vi "Teleop Operator Controls.vi"(7 "Call Context":T1=enum."Stop", 9 "Intaking":bool, 10 "Driver Agree To Shoot? (F)":bool, 11 "Match Info":T2={"Autonomous Elapsed Seconds"=0.0, "TeleOp Elapsed Seconds"=5.101, "Disabled Elapsed Seconds"=19.516, "Visited Autonomous"=FALSE, "Visited TeleOp"=TRUE, "Visited Disabled"=TRUE, "Autonomous Settings"={"Autonomous Style"=enum."Independent", "VI Refnum"=refnum}}) -> (3 "Operator Ready To Shoot?":bool)   [LabVIEW 2019]
uses:
  <vilib>/Rock Robotics/WPI/DriverStation/WPI_DriverStationMatch Info.ctl
  <vilib>/Rock Robotics/WPI/DriverStation/WPI_DriverStationDerivedRobotMode.ctl
  Typedef/XBox Axis.ctl
  Typedef/XBox Buttons.ctl
  Typedef/XBox POV.ctl
  <vilib>/Rock Robotics/WPI/Utilities/WPI_GetSetVariantRefNum.vi
panel:
  in  "LL Jog Amount":dbl
  in  "Hood Jog Amount Fast":dbl=0.5
  in  "Fast Jog Degress/frame":dbl=1.0
  in  "Jog Holdtime (ms)":u32=300
  in  "270 Hood Angle":dbl
  in  "180 Hood Angle":dbl
  in  "90 Hood Angle":dbl=10.0
  in  "0 Hood Angle":dbl=20.0
  in  "270 Angle":dbl
  in  "180 Angle":dbl
  in  "90 Angle":dbl=90.0
  in  "0 Angle":dbl
  in  "Hood Jog Amount":dbl=0.5
  in  "Jog Degrees":dbl=1.0
  in  "WoD Deadband":dbl=0.3
  in  "WoD Speed Factor":dbl=0.4
  in  "Uptake Speed":dbl=1.0 format="%#_13g"
  in  "Shooter Shoot RPM":dbl=7000.0
  in  "Shooter Idle RPM":dbl=2000.0
  in  "Turret Stick Deadband":dbl=0.9
  # "0"
  # "TURRET"
  # "HOOD"
  # "Joystick"
  # "90"
  # "270"
  # "180"
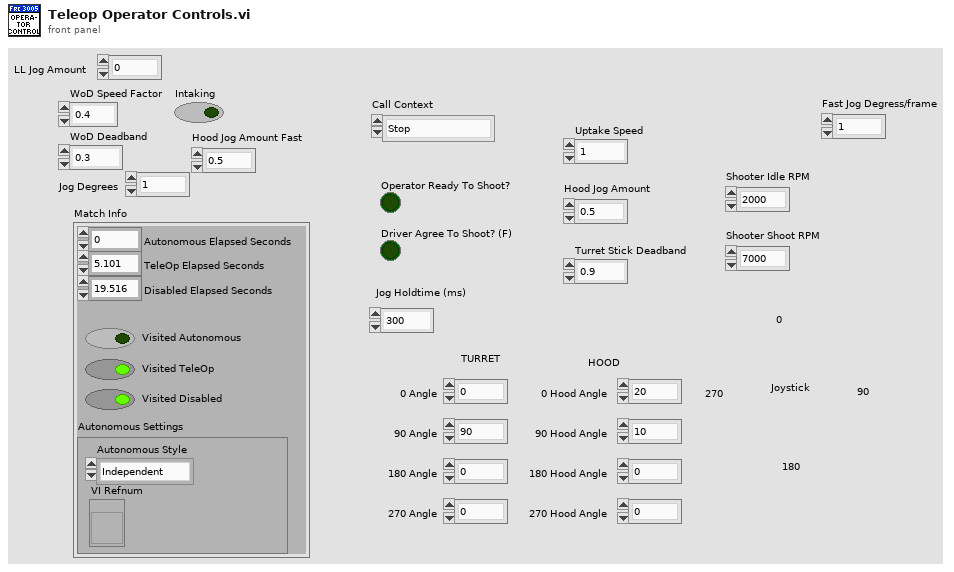
[diagram p1: front panel]
types:
  T1 = typedef "WPI_DriverStationDerivedRobotMode.ctl" = enum16{"Init", "Execute", "Stop"}
  T2 = typedef "WPI_DriverStationMatch Info.ctl" = cluster{"Autonomous Elapsed Seconds":dbl, "TeleOp Elapsed Seconds":dbl, "Disabled Elapsed Seconds":dbl, "Visited Autonomous":bool, "Visited TeleOp":bool, "Visited Disabled":bool, "Autonomous Settings":cluster{"Autonomous Style":enum16{"Iterative", "Independent"}, "VI Refnum":refnum<vi>}}
  T3 = typedef "XBox Axis.ctl" = enum16{"Left X", "Left Y", "Left Trigger", "Right Trigger", "Right X", "Right Y"}
  T4 = typedef "XBox Buttons.ctl" = enum16{"A", "B", "X", "Y", "Left Bumper", "Right Bumper", "Back", "Start", "Left Joystick", "Right Joystick"}
  T5 = typedef "XBox POV.ctl" = enum16{"Center", "Top", "Top Right", "Center Right", "Bottom Right", "Bottom", "Bottom Left", "Center Left", "Top Left"}
  T6 = typedef "WPI_JoystickDevRef.ctl" = cluster{"Device":T7}
  T7 = typedef "WPI_JoystickDeviceEnum.ctl" = enum16{"USB 0", "USB 1", "USB 2", "USB 3", "USB 4", "USB 5"}
  T8 = typedef "Command Status Info.ctl" = cluster{"Name":string, "Status":T9, "notifier out":T10}
  T9 = typedef "Completion Status.ctl" = enum16{"Successful", "Aborted", "Incomplete"}
  T10 = typedef "Completion Notifier.ctl" = refnum<notifier>
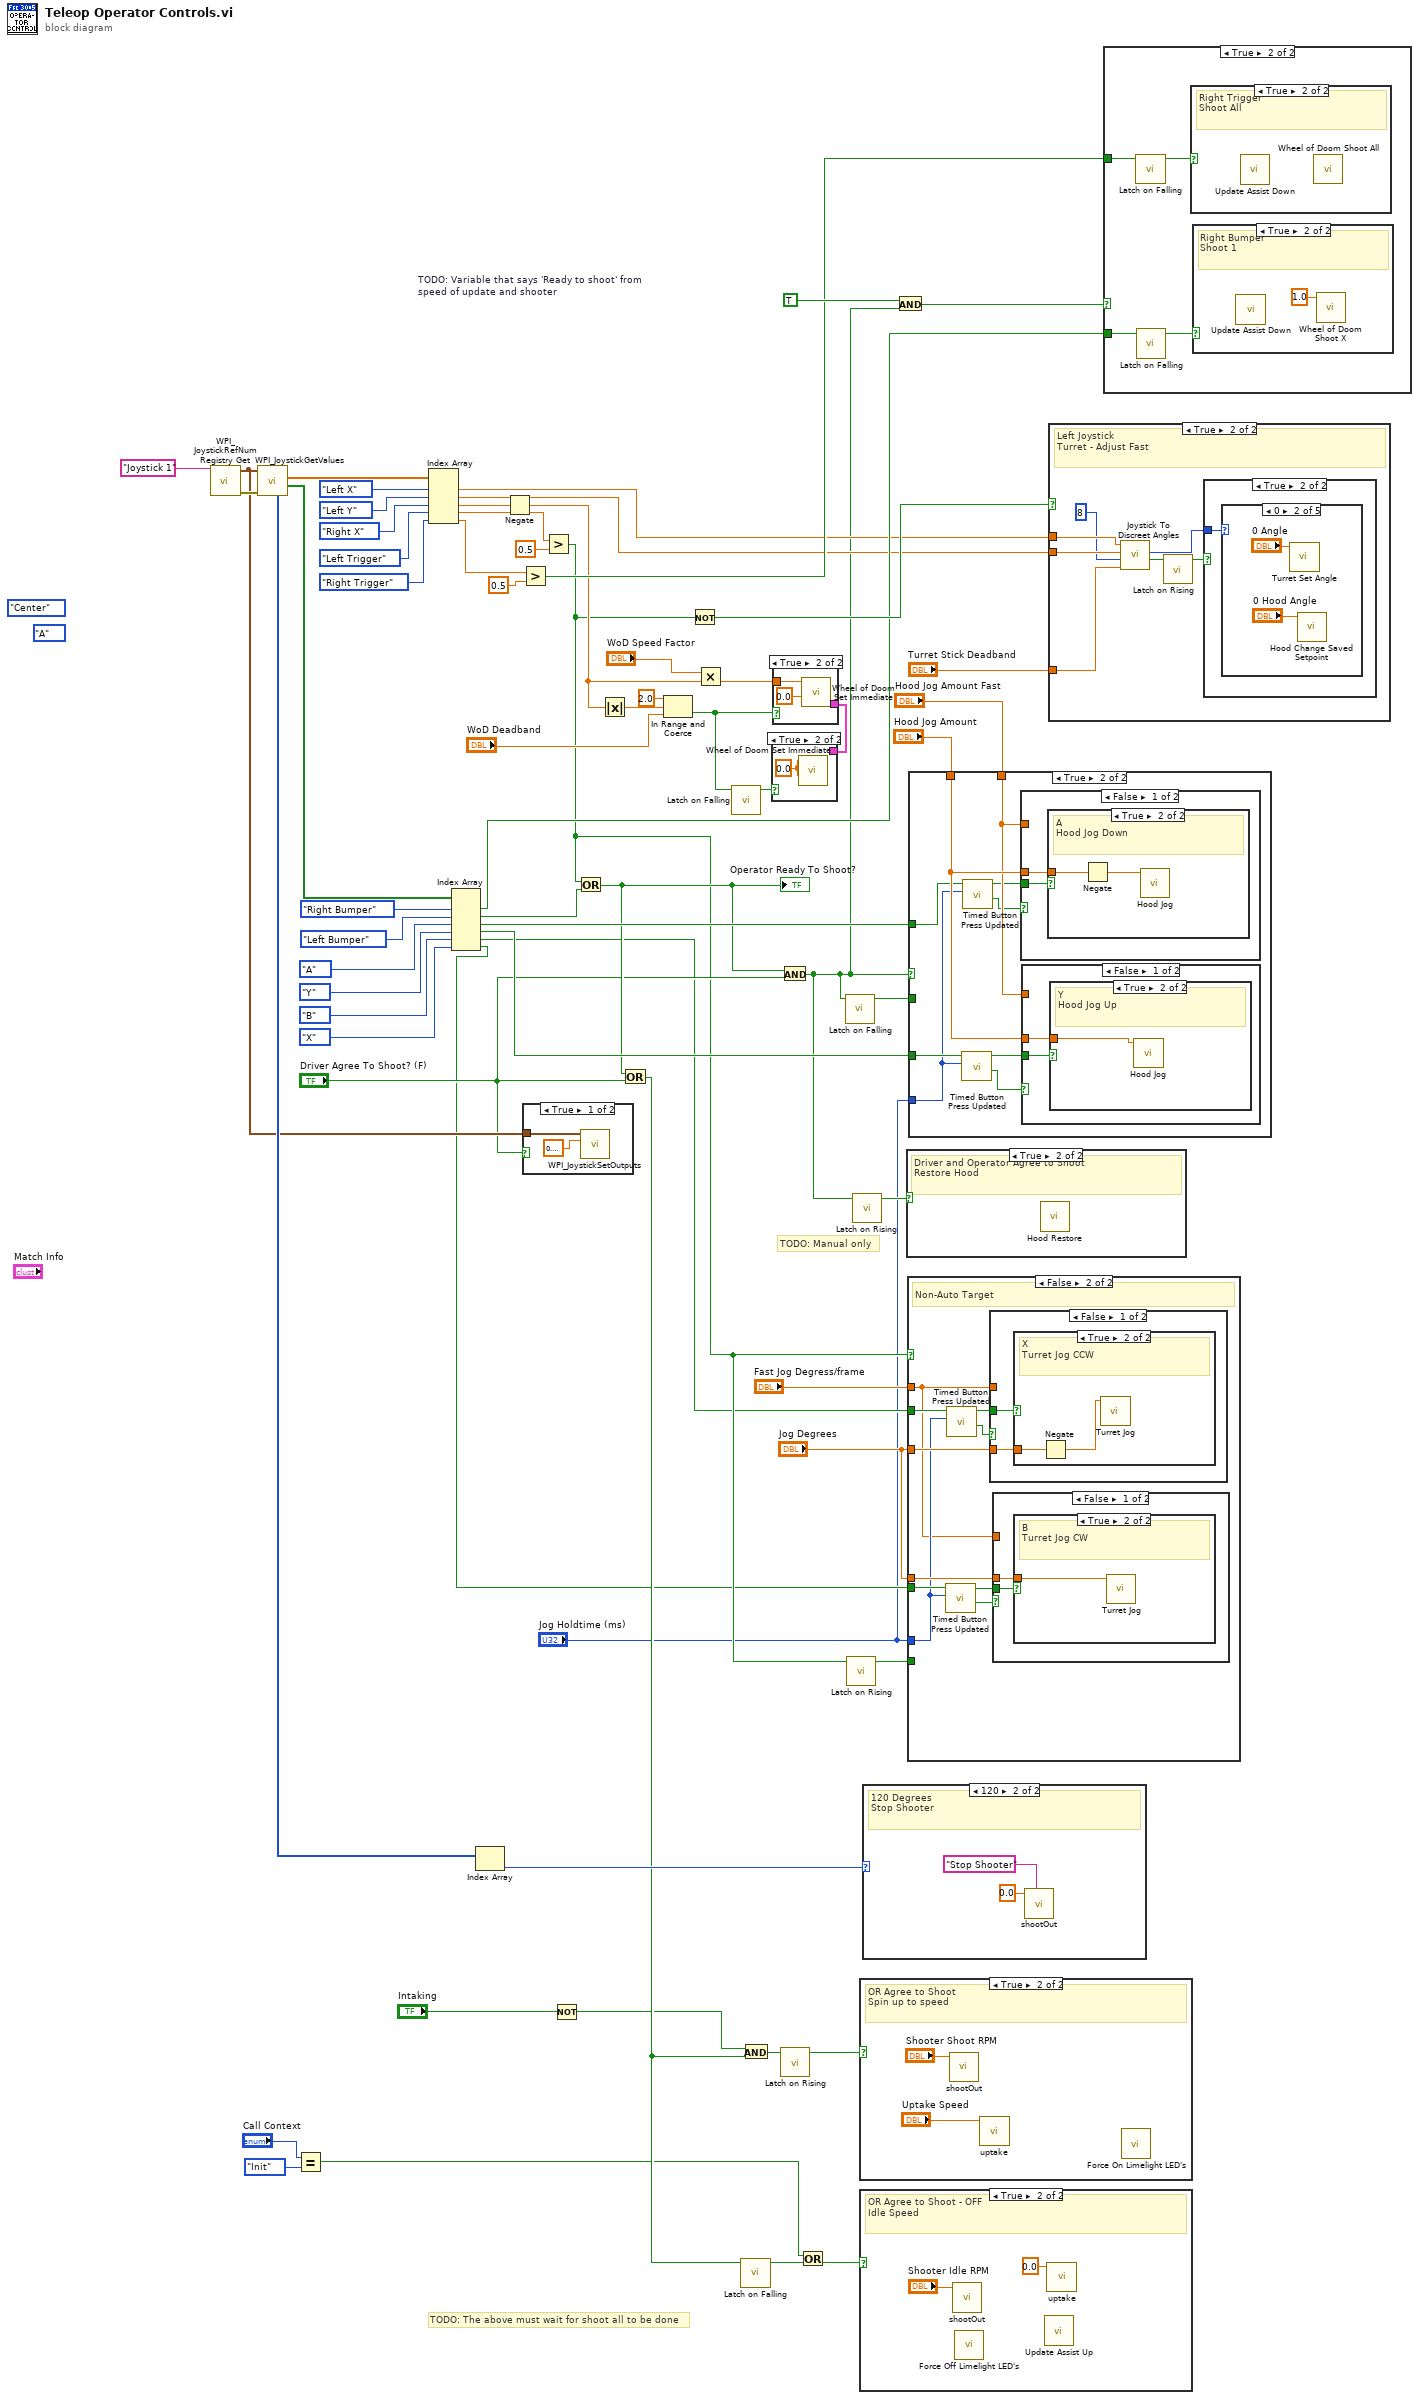
[diagram p0: block diagram]
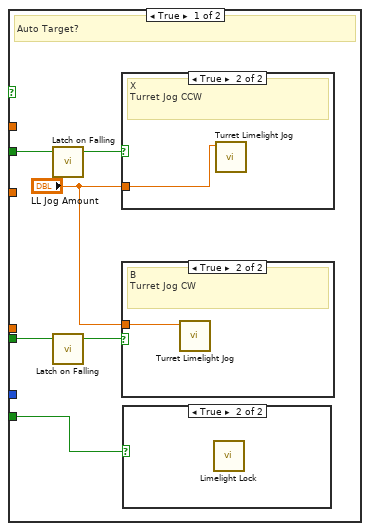
[diagram p3: hidden frame]
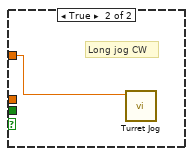
[diagram p8: hidden frame]
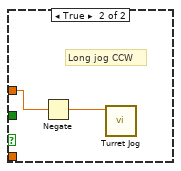
[diagram p10: hidden frame]
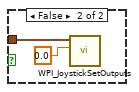
[diagram p11: hidden frame]
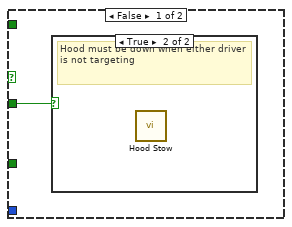
[diagram p19: hidden frame]
diagram:
  w44 = TRUE  # TODO: Variable that says 'Ready to shoot' from speed of update and shooter
  (unwired) XBox_Buttons."A" ("Enum 2")
  (unwired) XBox_POV."Center" ("Enum")
  # "TODO: Manual only"
  # "TODO: The above must wait for shoot all to be done"
  n1 = call <vilib>:"WPI_JoystickRefNum Registry Get.vi"("refnum name"="Joystick 1") -> ("error out"=w66:errorcluster, "JoystickDevRef"=w23:T6)  [unwired: 9 in]
  n2 = call <vilib>:"WPI_JoystickGetValues.vi"("error in (no error)"=w66, "JoystickDevRef"=w23) -> ("Buttons"=w64:bool[], "Axes"=w65:dbl[], "POVs"=w54:i16[])  [unwired: 5 in, 2 out]
  n3 = Equal?(x="Call Context", y=WPI_DriverStationDerivedRobotMode."Init") -> (x = y?=w8:bool)
  n4 = Index Array(array=w65, index #1=XBox_Axis."Left X" ("Enum 3"), index #2=XBox_Axis."Left Y" ("Enum 3"), index #3=XBox_Axis."Right X" ("Enum 3"), index #4=XBox_Axis."Left Trigger" ("Enum 3"), index #5=XBox_Axis."Right Trigger" ("Enum 3")) -> (element #1=w34:dbl, element #2=w33:dbl, element #3=w28:dbl, element #4=w50:dbl, element #5=w40:dbl)
  n5 = Index Array(array=w64, index #1=XBox_Buttons."Right Bumper" ("Enum 2"), index #2=XBox_Buttons."Left Bumper" ("Enum 2"), index #3=XBox_Buttons."A" ("Enum 2"), index #4=XBox_Buttons."Y" ("Enum 2"), index #5=XBox_Buttons."B" ("Enum 2"), index #6=XBox_Buttons."X" ("Enum 2")) -> (element #1=w42:bool, element #2=w48:bool, element #3=w61:bool, element #4=w56:bool, element #5=w7:bool, element #6=w6:bool)
  n6 = Index Array(array=w54) -> (element=w53:i16)  [unwired: 1 in]
  n7 = Negate(x=w28) -> (-x=w24:dbl)
  n8 = Greater?(x=w40, y=0.5) -> (0:w38:bool)
  n9 = case shown="True" "Driver Agree To Shoot? (F)" {
    tunnel: w23 -> [w69 w71]
    frame True {
      n10 = call <vilib>:"WPI_JoystickSetOutputs.vi"("Left Rumble"=sgl 0.3, "JoystickDevRef"=w69) -> ()  [unwired: 8 in, 2 out]
    }
    frame False {
      n11 = call <vilib>:"WPI_JoystickSetOutputs.vi"("Left Rumble"=sgl 0.0, "JoystickDevRef"=w71) -> ()  [unwired: 8 in, 2 out]
    }
  }
  n12 = Greater?(x=w50, y=0.5) -> (0:w19:bool)
  n13 = Not(x="Intaking") -> (.not. x?=w13:bool)
  n14 = Or(x=w19, y=w48) -> (x .or. y?=w37:bool)
  "Operator Ready To Shoot?" <- w37
  n15 = Absolute Value(x=w24) -> (abs(x)=w25:dbl)
  n16 = Or(x=w37, y="Driver Agree To Shoot? (F)") -> (x .or. y?=w15:bool)
  n17 = In Range and Coerce(upper limit=2.0, x=w25, lower limit="WoD Deadband") -> (In Range?=w27:bool)  [unwired: 1 out]
  n18 = Not(x=w19) -> (.not. x?=w46:bool)
  n19 = Multiply(x="WoD Speed Factor", y=w24) -> (x*y=w32:dbl)
  n20 = call <vilib>:"Latch on Falling.vi"("Boolean in"=w27) -> ("Boolean out"=w26:bool)  [unwired: 4 in]
  n21 = call <vilib>:"Latch on Falling.vi"("Boolean in"=w15) -> ("Boolean out"=w36:bool)  [unwired: 4 in]
  n22 = And(x=w13, y=w15) -> (x .and. y?=w16:bool)
  n23 = case shown="True" w27 {
    tunnel: w32 -> [_ w74]
    tunnel: [_ w72] -> w1
    frame False {
    }
    frame True {
      n24 = call "Wheel of Doom Set Immediate.vi"("Deadband Value"=0.0, "Setpoint"=w74) -> ("Command Info Out"=w72:T8)  [unwired: 9 in]
    }
  }
  n25 = case shown="True" w26 {
    tunnel: w1 -> [_ _]
    frame False {
    }
    frame True {
      w75 = 0.0 ("Deadband Value")
      n26 = call "Wheel of Doom Set Immediate.vi"("Deadband Value"=w75, "Setpoint"=w75) -> ()  [unwired: 9 in, 1 out]
    }
  }
  n27 = And(x=w37, y="Driver Agree To Shoot? (F)") -> (x .and. y?=w2:bool)
  n28 = call <vilib>:"Latch on Rising.vi"("Boolean in"=w16) -> ("Boolean out"=w35:bool)  [unwired: 4 in]
  n29 = Or(x=w8, y=w36) -> (x .or. y?=w11:bool)
  n30 = call <vilib>:"Latch on Falling.vi"("Boolean in"=w2) -> ("Boolean out"=w47:bool)  [unwired: 4 in]
  n31 = call <vilib>:"Latch on Rising.vi"("Boolean in"=w19) -> ("Boolean out"=w18:bool)  [unwired: 4 in]
  n32 = call <vilib>:"Latch on Rising.vi"("Boolean in"=w2) -> ("Boolean out"=w17:bool)  [unwired: 4 in]
  n33 = case shown="True" w35 {
    frame False {
    }
    frame True {
      # "OR Agree to Shoot\nSpin up to speed"
      n34 = call "shootOut.vi"("Setpoint"="Shooter Shoot RPM") -> ()  [unwired: 10 in, 1 out]
      n35 = call "uptake.vi"("Setpoint"="Uptake Speed") -> ()  [unwired: 10 in, 1 out]
      n36 = call "Force On Limelight LED's.vi"() -> ()  [unwired: 10 in, 1 out]
    }
  }
  n37 = case shown="True" w11 {
    frame False {
    }
    frame True {
      # "OR Agree to Shoot - OFF\nIdle Speed"
      n38 = call "shootOut.vi"("Setpoint"="Shooter Idle RPM") -> ()  [unwired: 10 in, 1 out]
      n39 = call "Force Off Limelight LED's.vi"() -> ()  [unwired: 10 in, 1 out]
      n40 = call "Update Assist Up.vi"() -> ()  [unwired: 11 in, 1 out]
      n41 = call "uptake.vi"("Setpoint"=0.0) -> ()  [unwired: 10 in, 1 out]
    }
  }
  n42 = case shown="120" w53 {
    frame 0, Default {
    }
    frame 120 {
      # "120 Degrees\nStop Shooter"
      n43 = call "shootOut.vi"("Description"="Stop Shooter", "Setpoint"=0.0) -> ()  [unwired: 9 in, 1 out]
    }
  }
  n44 = And(x=w44, y=w2) -> (x .and. y?=w45:bool)
  n45 = case shown="True" w17 {
    frame False {
    }
    frame True {
      # "Driver and Operator Agree to Shoot\nRestore Hood"
      n46 = call "Hood Restore.vi"() -> ()  [unwired: 11 in, 1 out]
    }
  }
  n47 = case shown="False" w19 {
    tunnel: w7 -> [w87 w95]
    tunnel: w6 -> [w86 w97]
    tunnel: "Jog Degrees" -> [_ w99]
    tunnel: "Jog Degrees" -> [_ w98]
    tunnel: w18 -> [w85 _]
    tunnel: "Jog Holdtime (ms)" -> [_ w93]
    tunnel: "Fast Jog Degress/frame" -> [_ w92]
    frame True {
      # "Auto Target?"
      n48 = call <vilib>:"Latch on Falling.vi"("Boolean in"=w87) -> ("Boolean out"=w82:bool)  [unwired: 4 in]
      n49 = call <vilib>:"Latch on Falling.vi"("Boolean in"=w86) -> ("Boolean out"=w83:bool)  [unwired: 4 in]
      n50 = case shown="True" w82 {
        tunnel: "LL Jog Amount" -> [_ w89]
        frame False {
        }
        frame True {
          # "X\nTurret Jog CCW"
          n51 = call "Turret Limelight Jog.vi"("Jog Amount"=w89) -> ()  [unwired: 11 in]
        }
      }
      n52 = case shown="True" w83 {
        tunnel: "LL Jog Amount" -> [_ w88]
        frame False {
        }
        frame True {
          # "B\nTurret Jog CW"
          n53 = call "Turret Limelight Jog.vi"("Jog Amount"=w88) -> ()  [unwired: 11 in]
        }
      }
      n54 = case shown="True" w85 {
        frame False {
        }
        frame True {
          n55 = call "Limelight Lock.vi"() -> ()  [unwired: 11 in, 1 out]
        }
      }
    }
    frame False {
      # "Non-Auto Target"
      n56 = call "Timed Button Press Updated.vi"("Holdtime (ms)"=w93, "Input"=w97) -> ("Long Press Held"=w91:bool, "Quick Press"=w96:bool)  [unwired: 6 in, 2 out]
      n57 = call "Timed Button Press Updated.vi"("Holdtime (ms)"=w93, "Input"=w95) -> ("Long Press Held"=w90:bool, "Quick Press"=w94:bool)  [unwired: 6 in, 2 out]
      n58 = case shown="False" w90 {
        tunnel: w99 -> [w105 _]
        tunnel: w94 -> [w104 _]
        tunnel: w92 -> [_ w108]
        frame False {
          n59 = case shown="True" w104 {
            tunnel: w105 -> [_ w107]
            frame False {
            }
            frame True {
              # "X\nTurret Jog CCW"
              n60 = Negate(x=w107) -> (-x=w106:dbl)
              n61 = call "Turret Jog.vi"("Jog Degrees"=w106) -> ()  [unwired: 10 in, 1 out]
            }
          }
        }
        frame True {
          # "Long jog CCW"
          n62 = Negate(x=w108) -> (-x=w109:dbl)
          n63 = call "Turret Jog.vi"("Jog Degrees"=w109) -> ()  [unwired: 10 in, 1 out]
        }
      }
      n64 = case shown="False" w91 {
        tunnel: w98 -> [w101 _]
        tunnel: w96 -> [w100 _]
        tunnel: w92 -> [_ w103]
        frame False {
          n65 = case shown="True" w100 {
            tunnel: w101 -> [_ w102]
            frame False {
            }
            frame True {
              # "B\nTurret Jog CW"
              n66 = call "Turret Jog.vi"("Jog Degrees"=w102) -> ()  [unwired: 10 in, 1 out]
            }
          }
        }
        frame True {
          # "Long jog CW"
          n67 = call "Turret Jog.vi"("Jog Degrees"=w103) -> ()  [unwired: 10 in, 1 out]
        }
      }
    }
  }
  n68 = case shown="True" w2 {
    tunnel: w61 -> [_ w115]
    tunnel: w56 -> [_ w117]
    tunnel: w47 -> [w110 _]
    tunnel: "Hood Jog Amount" -> [_ w119]
    tunnel: "Hood Jog Amount Fast" -> [_ w118]
    tunnel: "Jog Holdtime (ms)" -> [_ w113]
    frame False {
      n69 = case shown="True" w110 {
        frame False {
        }
        frame True {
          # "Hood must be down when either driver is not targeting"
          n70 = call "Hood Stow.vi"() -> ()  [unwired: 11 in, 1 out]
        }
      }
    }
    frame True {
      n71 = call "Timed Button Press Updated.vi"("Holdtime (ms)"=w113, "Input"=w117) -> ("Long Press Held"=w112:bool, "Quick Press"=w116:bool)  [unwired: 6 in, 2 out]
      n72 = call "Timed Button Press Updated.vi"("Holdtime (ms)"=w113, "Input"=w115) -> ("Long Press Held"=w111:bool, "Quick Press"=w114:bool)  [unwired: 6 in, 2 out]
      n73 = case shown="False" w111 {
        tunnel: w114 -> [w125 _]
        tunnel: w119 -> [w124 _]
        tunnel: w118 -> [_ w129]
        frame False {
          n74 = case shown="True" w125 {
            tunnel: w124 -> [_ w127]
            frame False {
            }
            frame True {
              # "A\nHood Jog Down"
              n75 = Negate(x=w127) -> (-x=w126:dbl)
              n76 = call "Hood Jog.vi"("Setpoint"=w126) -> ()  [unwired: 10 in, 1 out]
            }
          }
        }
        frame True {
          # "Jog while Holding"
          n77 = Negate(x=w129) -> (-x=w128:dbl)
          n78 = call "Hood Jog.vi"("Setpoint"=w128) -> ()  [unwired: 10 in, 1 out]
        }
      }
      n79 = case shown="False" w112 {
        tunnel: w116 -> [w121 _]
        tunnel: w119 -> [w120 _]
        tunnel: w118 -> [_ w123]
        frame False {
          n80 = case shown="True" w121 {
            tunnel: w120 -> [_ w122]
            frame False {
            }
            frame True {
              # "Y\nHood Jog Up"
              n81 = call "Hood Jog.vi"("Setpoint"=w122) -> ()  [unwired: 10 in, 1 out]
            }
          }
        }
        frame True {
          # "Jog while Holding"
          n82 = call "Hood Jog.vi"("Setpoint"=w123) -> ()  [unwired: 10 in, 1 out]
        }
      }
    }
  }
  n83 = case shown="True" w46 {
    tunnel: w34 -> [_ w136]
    tunnel: w33 -> [_ w135]
    tunnel: "Turret Stick Deadband" -> [_ w133]
    frame False {
    }
    frame True {
      # "Left Joystick\nTurret - Adjust Fast"
      n84 = call "Joystick To Discreet Angles.vi"("Deadband"=w133, "Zones"=8, "Y"=w135, "X"=w136) -> ("Valid"=w132:bool, "Discreet Angle"=w130:i32)  [unwired: 5 in, 1 out]
      n85 = call <vilib>:"Latch on Rising.vi"("Boolean in"=w132) -> ("Boolean out"=w131:bool)  [unwired: 4 in]
      n86 = case shown="True" w131 {
        tunnel: w130 -> [_ w137]
        frame False {
        }
        frame True {
          n87 = case shown="0" w137 {
            frame Default {
            }
            frame 0 {
              n88 = call "Turret Set Angle.vi"("Angle (Degrees)"="0 Angle") -> ()  [unwired: 10 in, 1 out]
              n89 = call "Hood Change Saved Setpoint.vi"("Setpoint"="0 Hood Angle") -> ()  [unwired: 10 in, 1 out]
            }
            frame 90 {
              n90 = call "Hood Change Saved Setpoint.vi"("Setpoint"="90 Hood Angle") -> ()  [unwired: 10 in, 1 out]
              n91 = call "Turret Set Angle.vi"("Angle (Degrees)"="90 Angle") -> ()  [unwired: 10 in, 1 out]
            }
            frame 180 {
              n92 = call "Turret Set Angle.vi"("Angle (Degrees)"="180 Angle") -> ()  [unwired: 10 in, 1 out]
              n93 = call "Hood Change Saved Setpoint.vi"("Setpoint"="180 Hood Angle") -> ()  [unwired: 10 in, 1 out]
            }
            frame 270 {
              n94 = call "Hood Change Saved Setpoint.vi"("Setpoint"="270 Hood Angle") -> ()  [unwired: 10 in, 1 out]
              n95 = call "Turret Set Angle.vi"("Angle (Degrees)"="270 Angle") -> ()  [unwired: 10 in, 1 out]
            }
          }
        }
      }
    }
  }
  n96 = case shown="True" w45 {
    tunnel: w42 -> [_ w149]
    tunnel: w38 -> [_ w148]
    frame False {
    }
    frame True {
      n97 = call <vilib>:"Latch on Falling.vi"("Boolean in"=w148) -> ("Boolean out"=w147:bool)  [unwired: 4 in]
      n98 = call <vilib>:"Latch on Falling.vi"("Boolean in"=w149) -> ("Boolean out"=w146:bool)  [unwired: 4 in]
      n99 = case shown="True" w147 {
        frame False {
        }
        frame True {
          # "Right Trigger\nShoot All"
          n100 = call "Update Assist Down.vi"() -> ()  [unwired: 11 in, 1 out]
          n101 = call "Wheel of Doom Shoot All.vi"() -> ()  [unwired: 11 in, 1 out]
        }
      }
      n102 = case shown="True" w146 {
        frame False {
        }
        frame True {
          # "Right Bumper\nShoot 1"
          n103 = call "Update Assist Down.vi"() -> ()  [unwired: 11 in, 1 out]
          n104 = call "Wheel of Doom Shoot X.vi"("Number to Shoot"=1.0 ("Setpoint")) -> ()  [unwired: 10 in, 1 out]
        }
      }
    }
  }
